vi "FileIO-Open Dialog (multiple).vi"(7 "Default Folder":path, 8 "error in":errorcluster, 10 "pattern (all files)":string="*.ini", 11 "Start path":path) -> (0 "error out":errorcluster, 1 "cancelled":bool, 3 "Paths":path[](array[path]))   [LabVIEW 2020]
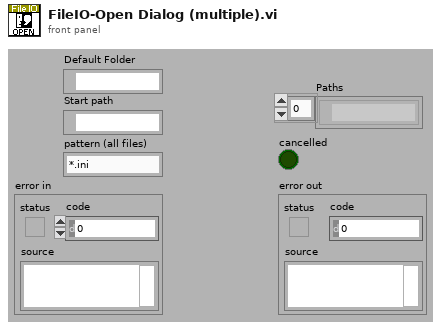
[diagram p1: front panel]
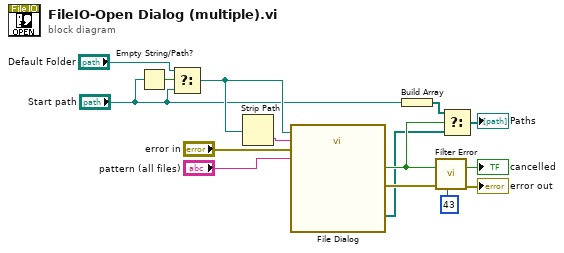
[diagram p0: block diagram]
diagram:
  n1 = Empty String/Path?(string/path="Start path") -> (empty?=w7:bool)
  n2 = Select(t="Default Folder", s=w7, f="Start path") -> (s? t:f=w5:path)
  n3 = Strip Path(path=w5) -> (name=w8:string)  [unwired: 1 out]
  n4 = call "File Dialog"("start path"=w5, "default name"=w8, "error in"="error in", "pattern (all files)"="pattern (all files)") -> ("selected paths"=w2:path[], "cancelled"=w9:bool, "error out"=w10:errorcluster)  [unwired: 8 in, 1 out]
  "cancelled" <- w9
  n5 = Build Array("Start path") -> (w3:path[])
  n6 = call "Filter Error.vi"("error in (no error)"=w10, "code to ignore"=43) -> ("error out"=→"error out":errorcluster)  [unwired: 9 in]
  n7 = Select(t=w3, s=w9, f=w2) -> (s? t:f=→"Paths":path[])
